vi "MCSTopLevel.vi"   [LabVIEW 2014]
uses:
  <vilib>/Platform/TimedLoop/XDataNode/wakeup.ctl
  <vilib>/Platform/TimedLoop/XDataNode/XDNodeRunTimeDep.lvlib
  <vilib>/Platform/TimedLoop/XDataNode/nitl_modes.ctl
  <vilib>/Platform/TimedLoop/XDataNode/timing_clust.ctl
  <vilib>/Platform/TimedLoop/XDataNode/XDataNode.xnode
  <vilib>/rvi/DataTransferAndStorage/Container/XNode/niFpgaContainer.xnode
  <vilib>/rvi/DataTransferAndStorage/Handshake/Emulation/niFpgaHandshakeEmulation.vi
  MCSGlobalVars.vi
  DAC/Code/FPGA SPI_Globals.vi
  Controls/MCSstate.ctl
  Sequencer/sequencerGlobVars.vi
types:
  T1 = typedef "MCSstate.ctl" = enum16{"idle", "scanning", "done", "error"}
  T2 = typedef "XDNodeRunTimeDep.lvlib/timing_clust.ctl" = cluster{"Expected End [f-1]":u64, "Actual End [f-1]":u64, "Finished Late? [f-1]":bool, "Expected End [i-1]":u64, "Actual End [i-1]":u64, "Finished Late? [i-1]":bool, "Expected Start [i]":u64, "Actual Start [i]":u64, "Expected Start [f]":u64, "Actual Start [f]":u64, "Source Name":string, "Structure Name":string, "Period":i64, "Deadline":i64, "Offset":i64, "Start":i64, "Priority":i32, "Timeout":i32, "Mode":T3, "Wakeup Reason":T4, "Error":errorcluster, "Source Type":string, "Secondary Source Type":string, "Global End Time":u64, "Global Start Time":u64, "Frame Duration":u64, "Iteration Duration":u64, "Assigned CPU":i32, "I/O Scan Engine Mode":u32}
  T3 = typedef "XDNodeRunTimeDep.lvlib/nitl_modes.ctl" = enum32{"No Change", "Process missed periods, maintain original phase", "Discard missed periods, maintain original phase", "Process missed periods, ignore original phase", "Discard missed periods, ignore original phase"}
  T4 = typedef "XDNodeRunTimeDep.lvlib/wakeup.ctl" = enum32{"Normal", "Aborted", "Asynchronous wakeup", "Timing source error", "Timed loop error", "Timeout"}
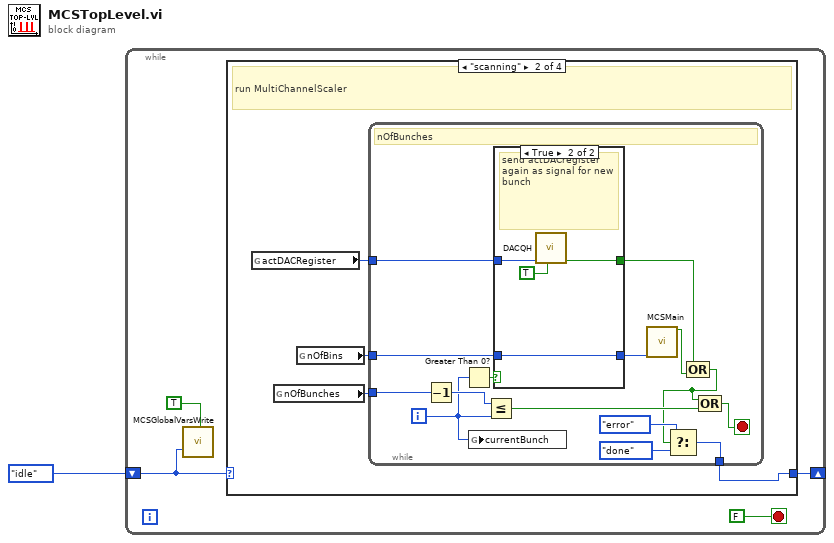
[diagram p0: block diagram]
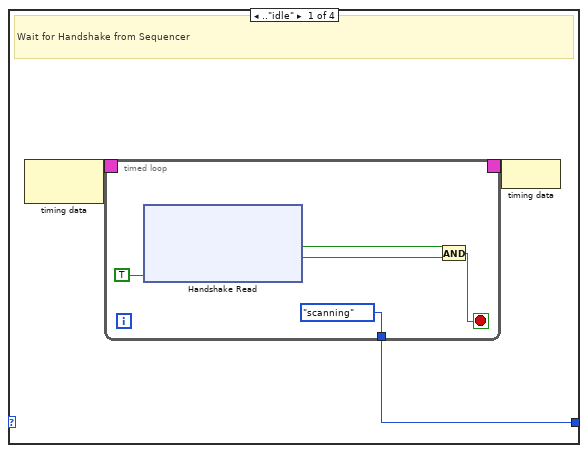
[diagram p2: hidden frame]
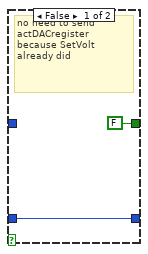
[diagram p3: hidden frame]
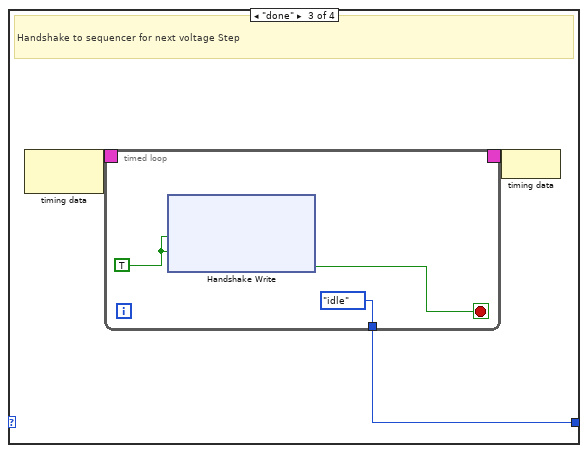
[diagram p4: hidden frame]
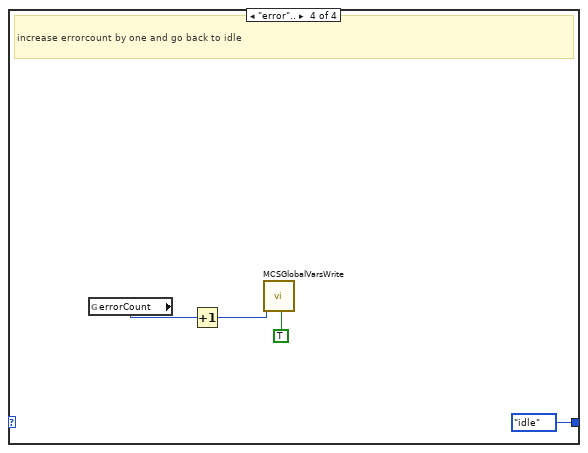
[diagram p5: hidden frame]
diagram:
  n1 = while {
    shift-right: [w4] -> _
    shift-left: MCSstate."idle" ("MCSstate") -> [w3]
    stop <- FALSE stop-if-true
    n2 = call "MCSGlobalVarsWrite.vi"("MCSstate"=w3, "writeOnlyMCSState"=TRUE) -> ()  [unwired: 18 in]
    n3 = case shown="\"scanning\"" w3 {
      tunnel: [w6 w18 w43 MCSstate."idle" ("MCSstate")] -> w4
      frame .."idle" {
        # "Wait for Handshake from Sequencer"
        n4 = node-c288() -> (w8:T2)  [unwired: 1 in]
        n5 = timed-loop {
          timing: w8 -> [_]
          timing-out: [_] -> w7
          tunnel: [MCSstate."scanning" ("MCSstate")] -> w6
          stop <- w10 stop-if-true
          n6 = xnode ("Handshake Read")("Ready for Output"=TRUE) -> ("Data"=w12:bool, "Output Valid"=w11:bool)  [unwired: 1 in, 1 out]
          n7 = And(x=w12, y=w11) -> (x .and. y?=w10:bool)
        }
        n8 = node-c288(w7) -> ()
      }
      frame "scanning" {
        # "run MultiChannelScaler"
        n9 = global read "FPGA SPI_Globals.vi" "actDACRegister"() -> (w19:u32)
        n10 = global read "MCSGlobalVars.vi" "nOfBunches"() -> (w20:i32)
        n11 = global read "MCSGlobalVars.vi" "nOfBins"() -> (w21:u32)
        n12 = while {
          tunnel: w20 -> [w35]
          tunnel: w21 -> [w31]
          tunnel: w19 -> [w33]
          tunnel: [w26] -> w18
          i -> [w22]
          stop <- w23 stop-if-true
          # "nOfBunches"
          n13 = Decrement(x=w35) -> (x-1=w36:i32)
          n14 = Greater Than 0?(x=w22) -> (x > 0?=w32:bool)
          n15 = global write "sequencerGlobVars.vi" "currentBunch"(w22) -> ()
          n16 = Less Or Equal?(x=w36, y=w22) -> (x <= y?=w27:bool)
          n17 = case shown="True" w32 {
            tunnel: w33 -> [_ w42]
            tunnel: w31 -> [w37 w41]
            tunnel: [w37 w41] -> w30
            tunnel: [FALSE ("DACQuWriteTimeout") w39] -> w29
            frame False {
              # "no need to send actDACregister because SetVolt already did"
            }
            frame True {
              # "send actDACregister again as signal for new bunch"
              n18 = call "DACQH.vi"("writeEqualsRead?"=TRUE, "Readback"=w42) -> ("DACQuWriteTimeout"=w39:bool)  [unwired: 9 in]
            }
          }
          n19 = call "MCSMain.vi"("nOfBins"=w30) -> ("abortOrTimeOut"=w34:bool)  [unwired: 18 in]
          n20 = Compound Arithmetic op=OR(w29, w34) -> (w25:bool)
          n21 = Select(t=MCSstate."error" ("MCSstate"), s=w25, f=MCSstate."done") -> (s? t:f=w26:T1)
          n22 = Compound Arithmetic op=OR(w25, w27) -> (w23:bool)
        }
      }
      frame "done" {
        # "Handshake to sequencer for next voltage Step"
        n23 = node-c288() -> (w45:T2)  [unwired: 1 in]
        n24 = timed-loop {
          timing: w45 -> [_]
          timing-out: [_] -> w44
          tunnel: [MCSstate."idle" ("MCSstate")] -> w43
          stop <- w48 stop-if-true
          w47 = TRUE ("Ready for Output")
          n25 = xnode ("Handshake Write")("Data"=w47, "Input Valid"=w47) -> ("Ready for Input"=w48:bool)  [unwired: 1 in, 1 out]
        }
        n26 = node-c288(w44) -> ()
      }
      frame "error".. {
        # "increase errorcount by one and go back to idle"
        n27 = global read "MCSGlobalVars.vi" "errorCount"() -> (w55:i8)
        n28 = Increment(x=w55) -> (x+1=w53:i8)
        n29 = call "MCSGlobalVarsWrite.vi"("errorCount"=w53, "writeOnlyErrorCount"=TRUE) -> ()  [unwired: 18 in]
      }
    }
  }
